vi "Set Decimation.vi"(8 "error in (no error)":errorcluster, 10 "Decimation":u32, 11 "RP Instrument in":refnum<class "RP Instrument.lvclass">) -> (0 "error out":errorcluster, 3 "RP Instrument out":refnum<class "RP Instrument.lvclass">)   [LabVIEW 2016, in "RP Instrument.lvclass"]
uses:
  RP Instrument.lvclass
  RP Instrument.lvclass/RP Instrument.ctl
  RP Config Offsets.ctl
  RP Command.ctl
  RP Communicator/RP Communicator.lvclass
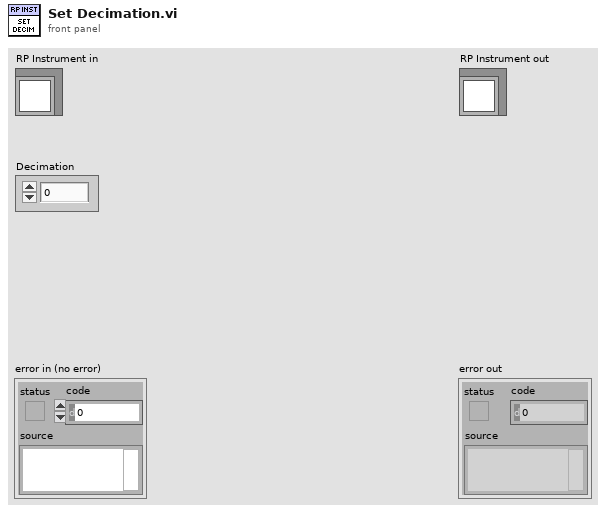
[diagram p1: front panel]
types:
  T1 = typedef "RP Command.ctl" = enum16{"Reset", "Read IDN", "Stop server", "Get status", "Get temperature", "Connect client", "Arm", "Software trigger", "Get whole buffer", "Get chunk", "System call", "Get config", "Set config", "Recieve data", "Recieve Calibartion", "Transmit data"}
  T2 = typedef "RP Config Offsets.ctl" = u16
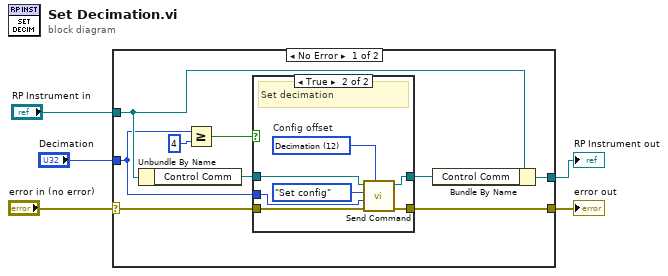
[diagram p0: block diagram]
diagram:
  n1 = case shown="No Error" "error in (no error)" {
    selector: "error in (no error)" -> [w11 w25]
    tunnel: [w10 w25] -> w4
    tunnel: [w14 w24] -> w2
    tunnel: "RP Instrument in" -> [w13 w24]
    tunnel: "Decimation" -> [w6 _]
    frame No Error {
      n2 = Unbundle By Name(w13) -> ("Control Comm"=w12:refnum<class "RP Communicator.lvclass">)
      n3 = Greater Or Equal?(x=w6, y=u32 4) -> (x >= y?=w7:bool)
      n4 = case shown="True" w7 {
        tunnel: w11 -> [w15 w23]
        tunnel: w12 -> [w16 w22]
        tunnel: [w15 w21] -> w10
        tunnel: [w16 w20] -> w9
        tunnel: w6 -> [_ w19]
        frame False {
        }
        frame True {
          w18 = T2 12 items=["Config flags"=0, "Record length"=4, "Frequency"=8, "Decimation"=12, "LED"=16]  # Config offset
          # "Set decimation"
          n5 = call-dynamic "Send Command.vi"("Config offset"=w18, "error in (no error)"=w23, "Command payload"=w19, "Command number"=RP_Command."Set config", "RP Communicator in"=w22) -> ("error out"=w21:errorcluster, "RP Communicator out"=w20:refnum<class "RP Communicator.lvclass">)  [unwired: 5 in]
        }
      }
      n6 = Bundle By Name(cluster=w13, "Control Comm"=w9) -> (w14:refnum<class "RP Instrument.lvclass">)
    }
    frame Error {
    }
  }
  "error out" <- w4
  "RP Instrument out" <- w2
